vi "Extract features.vi"(8 "Error In":errorcluster, 11 "Event cluster":T1) -> (0 "Error Out":errorcluster, 2 "Event features":dbl[](array[numeric]))   [LabVIEW 2016]
uses:
  Typedef/Event cluster.ctl
  Typedef/SVM train class.ctl
  Typedef/SVM predict class.ctl
  <vilib>/Analysis/NI_AALBase.lvlib
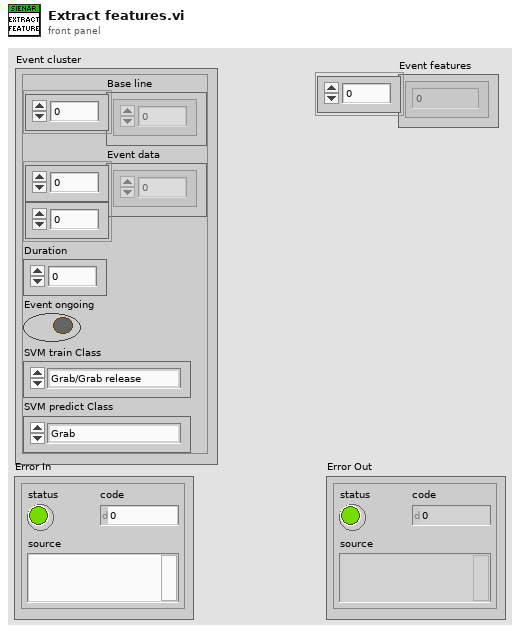
[diagram p1: front panel]
types:
  T1 = typedef "Event cluster.ctl" = cluster{"Base line":dbl[], "Event data":dbl[][], "Duration":dbl, "Event ongoing":bool, "SVM train Class":T2, "SVM predict Class":T3}
  T2 = typedef "SVM train class.ctl" = enum16{"Grab/Grab release", "Hand flexion/HF release", "Hand extension/HE release", "Tap", "Swipe_CW", "Swipe_CCW"}
  T3 = typedef "SVM predict class.ctl" = enum16{"Grab", "Grab release", "Hand flexion", "Hand flexion release", "Hand extension", "Hand extension release", "Tap", "Swipe_CW", "Swipe_CCW"}
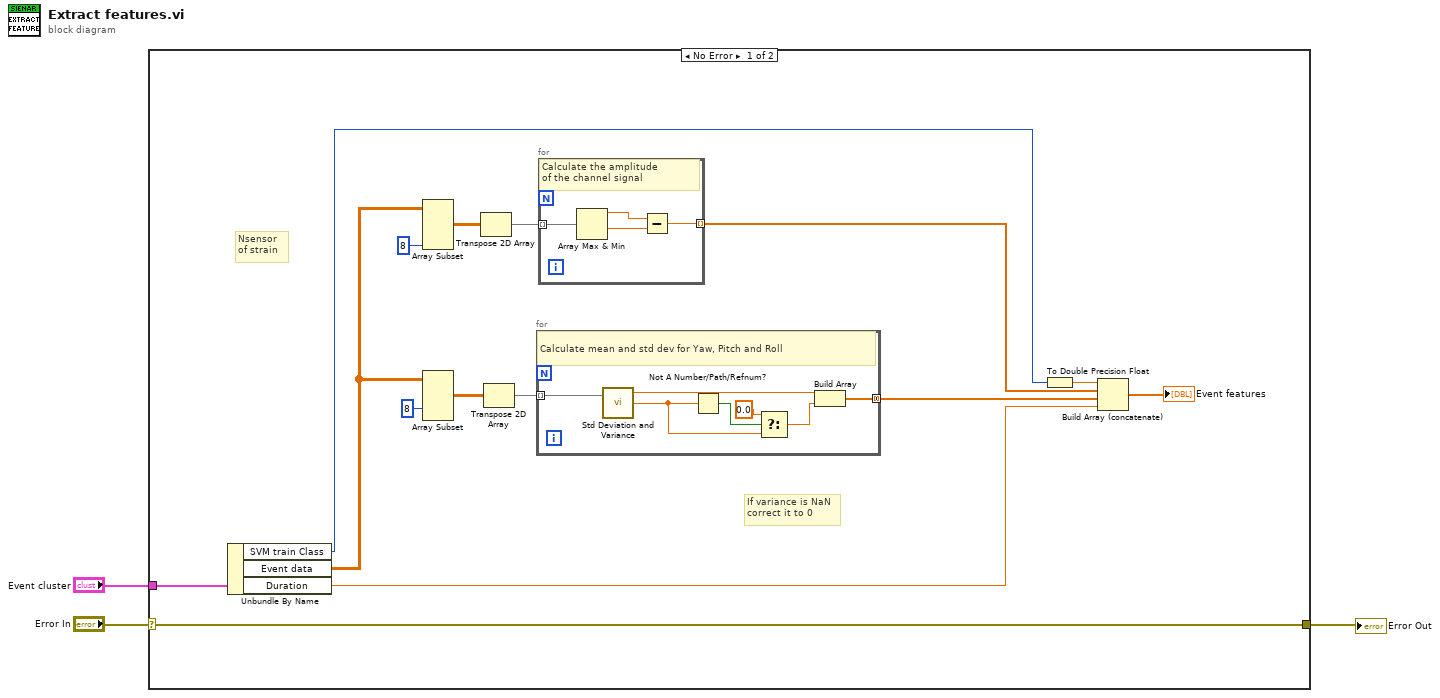
[diagram p0: block diagram]
diagram:
  n1 = case shown="No Error" "Error In" {
    selector: "Error In" -> [w18 w30]
    tunnel: [w18 w30] -> w2
    tunnel: "Event cluster" -> [w17 _]
    frame No Error {
      # "If variance is NaN\ncorrect it to 0"
      # "Nsensor\nof strain"
      n2 = Unbundle By Name(w17) -> ("SVM train Class"=w4:T2, "Event data"=w6:dbl[][], "Duration"=w11:dbl)
      n3 = Array Subset(array=w6, length (col)=8 ("index")) -> (w8:dbl[][])  [unwired: 3 in]
      n4 = Array Subset(array=w6, index (col)=8 ("index")) -> (w14:dbl[][])  [unwired: 3 in]
      n5 = Transpose 2D Array(2D array=w8) -> (transposed array=w9:dbl[][])
      n6 = Transpose 2D Array(2D array=w14) -> (transposed array=w15:dbl[][])
      n7 = for {
        tunnel: w15 -> [w25] mode=indexing
        tunnel: [w23] -> w12 mode=concatenating
        # "Calculate mean and std dev for Yaw, Pitch and Roll"
        n8 = call <vilib>:"Std Deviation and Variance.vi"("X"=w25) -> ("mean"=w24:dbl, "standard deviation"=w21:dbl)  [unwired: 1 in, 1 out]
        n9 = Not A Number/Path/Refnum?(number/path/refnum=w21) -> (NaN/Path/Refnum?=w22:bool)
        n10 = Select(t=0.0, s=w22, f=w21) -> (s? t:f=w20:dbl)
        n11 = Build Array(w24, w20) -> (w23:dbl[])
      }
      n12 = for {
        tunnel: w9 -> [w29] mode=indexing
        tunnel: [w26] -> w13 mode=indexing
        # "Calculate the amplitude\nof the channel signal"
        n13 = Array Max & Min(array=w29) -> (max value=w28:dbl, min value=w27:dbl)  [unwired: 2 out]
        n14 = Subtract(x=w28, y=w27) -> (x-y=w26:dbl)
      }
      n15 = To Double Precision Float(number=w4) -> (double precision float=w5:dbl)
      n16 = Build Array (concatenate)(w5, w13, w12, w11) -> (→"Event features":dbl[])
    }
    frame Error {
    }
  }
  "Error Out" <- w2
